vi "Change_value.vi"(8 "error in (no error)":errorcluster, 9 "Data string":string, 10 "Task name":string, 11 "DAQmxTaksContainer_General in":refnum<class "DAQmxTaksContainer_General.lvclass">) -> (0 "error out":errorcluster, 3 "DAQmxTaksContainer_General out":refnum<class "DAQmxTaksContainer_General.lvclass">)   [LabVIEW 2015, in "DAQmxTaksContainer_General.lvclass"]
uses:
  DAQmxTaksContainer_General.lvclass
  DAQmxTaksContainer_General.lvclass/DAQmxTaksContainer_General.ctl
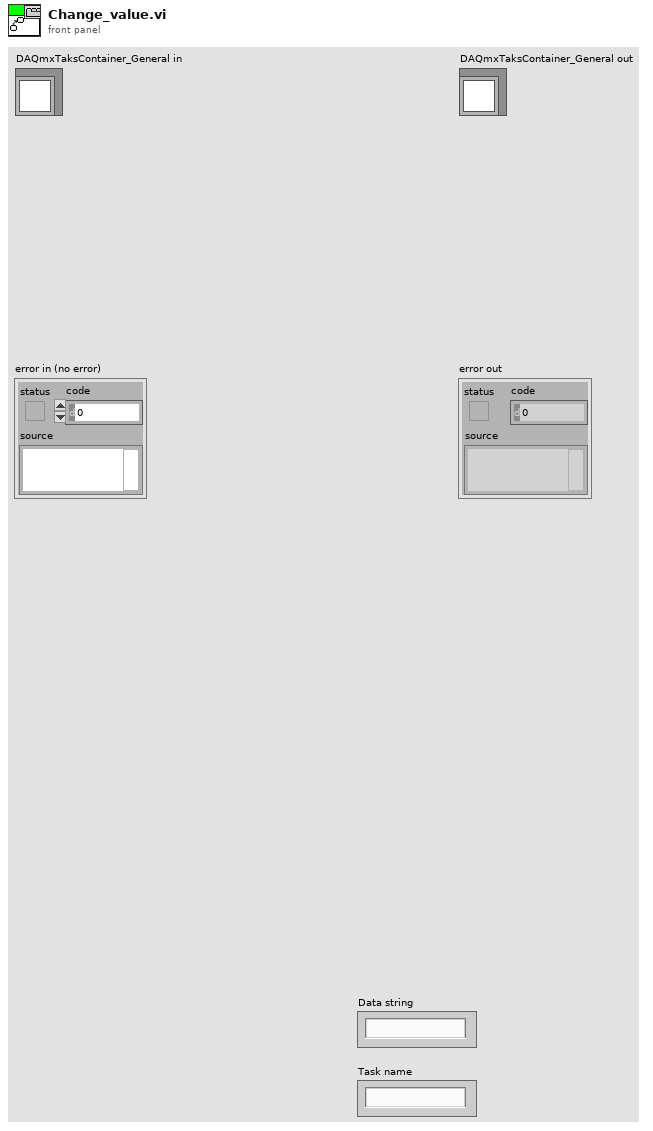
[diagram p1: front panel]
types:
  T1 = cluster{"name":string, "type of task":string, "Status":bool, "Value":string, "error":errorcluster}[]
  T2 = cluster{"name":string, "type of task":string, "Status":bool, "Value":string, "error":errorcluster}
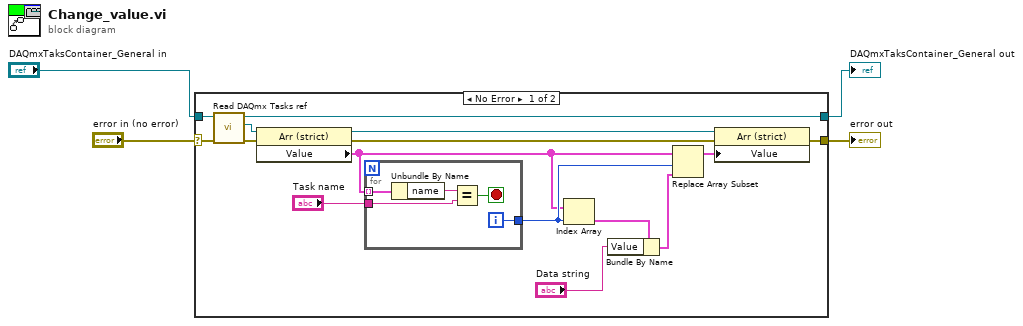
[diagram p0: block diagram]
diagram:
  n1 = case shown="No Error" "error in (no error)" {
    selector: "error in (no error)" -> [w13 w26]
    tunnel: [w6 w26] -> w3
    tunnel: [w5 w25] -> w1
    tunnel: "DAQmxTaksContainer_General in" -> [w14 w25]
    frame No Error {
      n2 = call "Read DAQmx Tasks ref.vi"("error in (no error)"=w13, "DAQmxTaksContainer_General in"=w14) -> ("error out"=w11:errorcluster, "DAQmx Tasks ref"=w12:refnum<vi>, "DAQmxTaksContainer_General out"=w5:refnum<class "DAQmxTaksContainer_General.lvclass">)  [unwired: 7 in]
      n3 = property class="Arr (strict)"(reference=w12, error in=w11) -> (reference out=w7:refnum<vi>, error out=w8:errorcluster, "Value"=w9:T1)
      n4 = for {
        tunnel: w9 -> [w20] mode=indexing
        tunnel: "Task name" -> [w23]
        tunnel: [w21] -> w17
        i -> [w21]
        stop <- w22 stop-if-true
        n5 = Unbundle By Name(w20) -> ("name"=w24:string)
        n6 = Equal?(x=w24, y=w23) -> (x = y?=w22:bool)
      }
      n7 = Index Array(array=w9, index=w17) -> (element=w18:T2)
      n8 = Bundle By Name(cluster=w18, "Value"="Data string") -> (w16:T2)
      n9 = Replace Array Subset(array=w9, new element=w16, index=w17) -> (w10:T1)
      n10 = property class="Arr (strict)"(reference=w7, error in=w8, "Value"=w10) -> (error out=w6:errorcluster)  [unwired: 1 out]
    }
    frame Error {
    }
  }
  "error out" <- w3
  "DAQmxTaksContainer_General out" <- w1
